vi "Read Event.vi"(8 "error in (no error)":errorcluster caption="entrée d'erreur (pas d'erreur)", 11 "Class Event Shielding Box en entrée":refnum<class "Class Event DIO.lvclass">) -> (0 "error out":errorcluster caption="sortie d'erreur", 3 "Class Event Shielding Box en sortie":refnum<class "Class Event DIO.lvclass">)   [LabVIEW 2020, in "Library Instrument & Equipement.lvlib" / "Library Event.lvlib" / "Class Event DIO.lvclass"]
uses:
  Class Event DIO.lvclass
  C:/Users/ngarcin/OneDrive - Altyor/Standard TB/Class/Core/Actors/Actor_EventStart/Classe Event (Default)/Class Event (Default).lvclass
  Commun VI/TypeDef/Commande DIO/Parameter DIO.ctl
  DIO/Class DIO (Default)/Class DIO (Default).lvclass
  JSON API/JSON Value/Set from JSON string.vi
  JSON API/Variant JSON/Variant to JSON.vi
  JSON API/JSON Value/Get Item by name array.vi
  Instrument/Instrument (Default)/Class Instrument (Default).lvclass
  JSON API/JSON Value/JSON Value.lvclass
  Class Event DIO.lvclass/Class Event DIO.ctl
  JSON API/Variant JSON/Variant JSON.lvlib
  JSON API/Get Polymorphic/JSON GetSet.lvlib
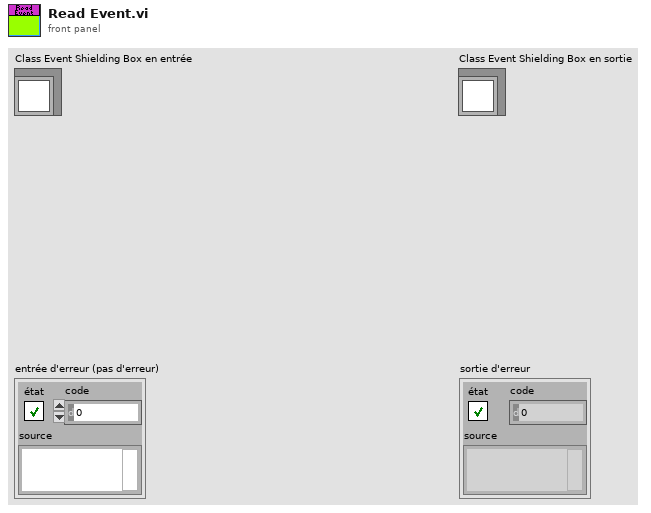
[diagram p1: front panel]
types:
  T1 = typedef "Parameter DIO.ctl" = cluster{"Device_Com_Port":string, "Port":u8, "Line":u8, "Function":enum16{"Write", "Read"}, "Class DIO":refnum<class "Class DIO (Default).lvclass">}
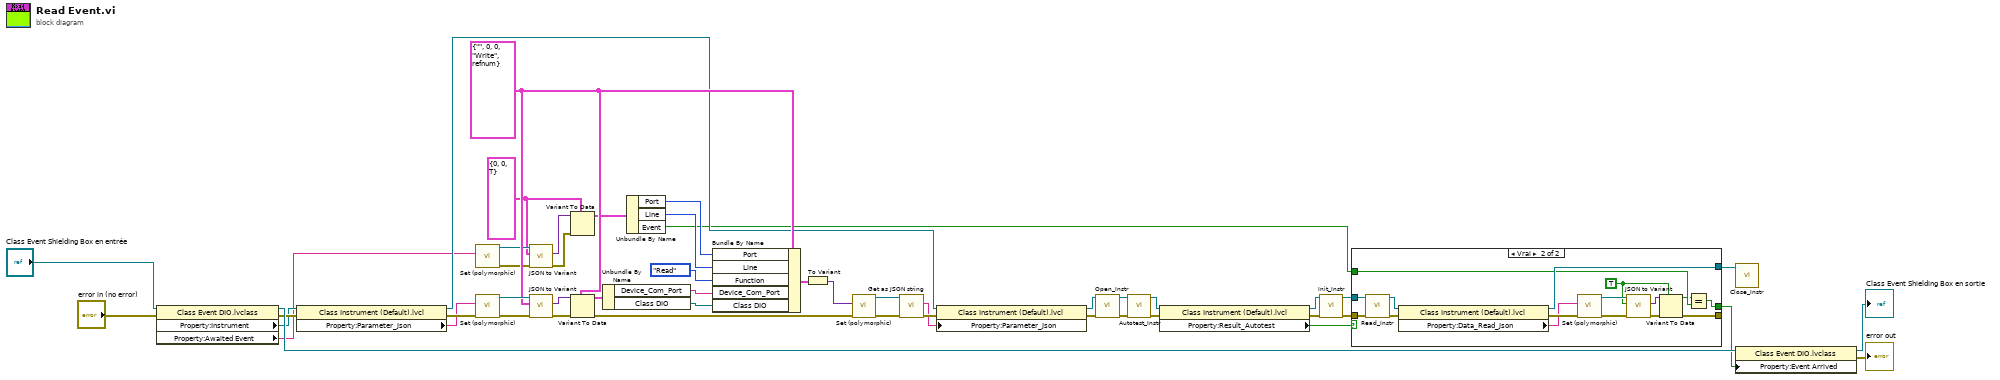
[diagram p0: block diagram]
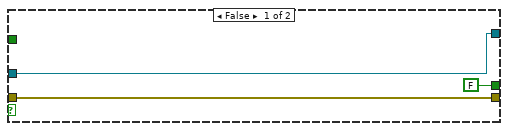
[diagram p2: hidden frame]
diagram:
  w5 = cluster{"Line":u8, "Port":u8, "Event":bool} {"Line"=0, "Port"=0, "Event"=TRUE}
  w27 = T1 {"Device_Com_Port"="", "Port"=0, "Line"=0, "Function"=enum."Write", "Class DIO"=refnum} ("Parameter")
  n1 = property class="Class Event DIO.lvclass"(reference="Class Event Shielding Box en entrée", error in="error in (no error)") -> (reference out=w41:refnum<class "Class Event DIO.lvclass">, error out=w19:errorcluster, "Property:Instrument"=w18:refnum<class "Class Instrument (Default).lvclass">, "Property:Awaited Event"=w6:string)
  n2 = property class="Class Instrument (Default).lvcl"(reference=w18, error in=w19) -> (reference out=w21:refnum<class "Class Instrument (Default).lvclass">, error out=w26:errorcluster, "Property:Parameter_Json"=w22:string)
  n3 = call-poly "Set (polymorphic).vi"("JSON stream"=w6) -> ("error out"=w9:errorcluster, "JSON Value out"=w11:refnum<class "JSON Value.lvclass">)  [unwired: 8 in, 1 out]
  n4 = call-poly "Set (polymorphic).vi"("error in (no error)"=w26, "JSON stream"=w22) -> ("error out"=w30:errorcluster, "JSON Value out"=w28:refnum<class "JSON Value.lvclass">)  [unwired: 7 in, 1 out]
  n5 = call "JSON to Variant.vi"("error in (no error)"=w9, "Variant (Data Type)"=w5, "JSON Value"=w11) -> ("error out"=w10:errorcluster, "Variant out"=w8:variant)  [unwired: 7 in]
  n6 = call "JSON to Variant.vi"("error in (no error)"=w30, "Variant (Data Type)"=w27, "JSON Value"=w28) -> ("error out"=w29:errorcluster, "Variant out"=w31:variant)  [unwired: 7 in]
  n7 = Variant To Data(error in=w10, type=w5, Variant=w8) -> (data=w7:cluster{"Line":u8, "Port":u8, "Event":bool})  [unwired: 1 out]
  n8 = Variant To Data(error in=w29, type=w27, Variant=w31) -> (data=w24:T1, error out=w25:errorcluster)
  n9 = Unbundle By Name(w24) -> ("Device_Com_Port"=w23:string, "Class DIO"=w20:refnum<class "Class DIO (Default).lvclass">)
  n10 = Unbundle By Name(w7) -> ("Port"=w14:u8, "Line"=w13:u8, "Event"=w12:bool)
  n11 = Bundle By Name(cluster=w27, "Port"=w14, "Line"=w13, "Function"=enum16{"Write", "Read"}."Read", "Device_Com_Port"=w23, "Class DIO"=w20) -> (w33:T1)
  n12 = To Variant(anything=w33) -> (Variant=w37:variant)
  n13 = call-poly "Set (polymorphic).vi"("error in (no error)"=w25, "Variant"=w37) -> ("error out"=w35:errorcluster, "JSON Value out"=w36:refnum<class "JSON Value.lvclass">)  [unwired: 8 in]
  n14 = call "Get as JSON string.vi"("error in (no error)"=w35, "JSON Value in"=w36) -> ("error out"=w34:errorcluster, "<JSON>"=w32:string)  [unwired: 8 in]
  n15 = property class="Class Instrument (Default).lvcl"(reference=w21, error in=w34, "Property:Parameter_Json"=w32) -> (reference out=w17:refnum<class "Class Instrument (Default).lvclass">, error out=w16:errorcluster)
  n16 = call-dynamic "Open_Instr.vi"("error in (no error)"=w16, "Class Multimeter (Default) en entrée"=w17) -> ("error out"=w43:errorcluster, "Class Multimeter (Default) en sortie"=w47:refnum<class "Class Instrument (Default).lvclass">)  [unwired: 8 in]
  n17 = call-dynamic "Autotest_Instr.vi"("error in (no error)"=w43, "Class Instrument (Default) en entrée"=w47) -> ("error out"=w44:errorcluster, "Class Instrument (Default) en sortie"=w46:refnum<class "Class Instrument (Default).lvclass">)  [unwired: 8 in]
  n18 = property class="Class Instrument (Default).lvcl"(reference=w46, error in=w44) -> (reference out=w3:refnum<class "Class Instrument (Default).lvclass">, error out=w2:errorcluster, "Property:Result_Autotest"=w45:bool)
  n19 = call-dynamic "Init_Instr.vi"("error in (no error)"=w2, "Class Instrument (Default) en entrée"=w3) -> ("error out"=w1:errorcluster, "Class Instrument (Default) en sortie"=w4:refnum<class "Class Instrument (Default).lvclass">)  [unwired: 8 in]
  n20 = case shown="Vrai" w45 {
    tunnel: w1 -> [w51 w68]
    tunnel: w4 -> [w52 w67]
    tunnel: [w52 w64] -> w42
    tunnel: [w51 w53] -> _
    tunnel: [FALSE w57] -> w38
    tunnel: w12 -> [_ w55]
    frame False {
    }
    frame True {
      w56 = TRUE
      n21 = call-dynamic "Read_Instr.vi"("error in (no error)"=w68, "Class Instrument (Default) en entrée"=w67) -> ("error out"=w65:errorcluster, "Class Instrument (Default) en sortie"=w66:refnum<class "Class Instrument (Default).lvclass">)  [unwired: 8 in]
      n22 = property class="Class Instrument (Default).lvcl"(reference=w66, error in=w65) -> (reference out=w64:refnum<class "Class Instrument (Default).lvclass">, error out=w59:errorcluster, "Property:Data_Read_Json"=w58:string)
      n23 = call-poly "Set (polymorphic).vi"("error in (no error)"=w59, "JSON stream"=w58) -> ("error out"=w62:errorcluster, "JSON Value out"=w60:refnum<class "JSON Value.lvclass">)  [unwired: 7 in, 1 out]
      n24 = call "JSON to Variant.vi"("error in (no error)"=w62, "Variant (Data Type)"=w56, "JSON Value"=w60) -> ("error out"=w61:errorcluster, "Variant out"=w63:variant)  [unwired: 7 in]
      n25 = Variant To Data(error in=w61, type=w56, Variant=w63) -> (data=w54:bool, error out=w53:errorcluster)
      n26 = Equal?(x=w54, y=w55) -> (x = y?=w57:bool)
    }
  }
  n27 = call-dynamic "Close_Instr.vi"("Class Instrument (Default) en entrée"=w42) -> ()  [unwired: 9 in, 2 out]
  n28 = property class="Class Event DIO.lvclass"(reference=w41, "Property:Event Arrived"=w38) -> (reference out=→"Class Event Shielding Box en sortie":refnum<class "Class Event DIO.lvclass">, error out=→"error out":errorcluster)  [unwired: 1 in]
